vi "Create PUBREC Packet.vi"(5 "PUBREC in":refnum<class "PUBREC.lvclass">, 8 "error in (no error)":errorcluster, 9 "Packet ID":u16 format="%04x") -> (0 "error out":errorcluster, 2 "Bytes Stream":u8[](array[numeric]) format="%08b", 3 "PUBREC out":refnum<class "PUBREC.lvclass">)   [LabVIEW 2013, in "MQTT_Control_Packets.lvlib" / "PUBREC.lvclass"]
uses:
  PUBREC.lvclass
  ControlPacket/ControlPacket.lvclass/ControlPacket.ctl
  ControlPacket/ControlPacket.lvclass
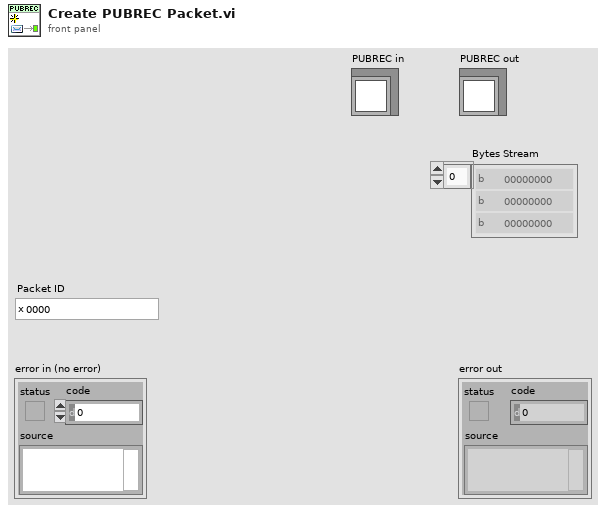
[diagram p1: front panel]
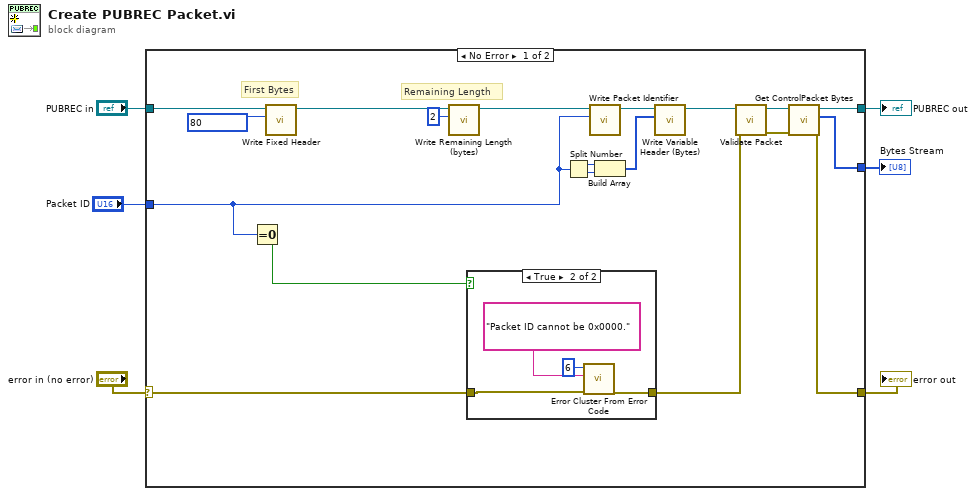
[diagram p0: block diagram]
diagram:
  n1 = case shown="No Error" "error in (no error)" {
    selector: "error in (no error)" -> [w13 w32]
    tunnel: [w9 w32] -> w3
    tunnel: [w7 w31] -> w4
    tunnel: "PUBREC in" -> [w25 w31]
    tunnel: "Packet ID" -> [w15 _]
    tunnel: [w11 _] -> w1
    frame No Error {
      # "Remaining Length"
      # "First Bytes"
      n2 = Equal To 0?(x=w15) -> (x = 0?=w14:bool)
      n3 = call "Write Fixed Header.vi"("Fixed Header"=u8 80, "ControlPacket in"=w25) -> ("ControlPacket out"=w24:refnum<class "PUBREC.lvclass">)  [unwired: 9 in]
      n4 = call "Write Remaining Length (bytes).vi"("Remaining Length (bytes)"=u32 2, "ControlPacket in"=w24) -> ("ControlPacket out"=w20:refnum<class "PUBREC.lvclass">)  [unwired: 9 in]
      n5 = case shown="True" w14 {
        tunnel: w13 -> [w26 w29]
        tunnel: [w26 w30] -> w12
        frame False {
        }
        frame True {
          n6 = call <vilib>:"Error Cluster From Error Code.vi"("error in (no error)"=w29, "error message (\"\")"="Packet ID cannot be 0x0000.", "error code (0)"=6) -> ("error out"=w30:errorcluster)  [unwired: 6 in]
        }
      }
      n7 = Split Number(x=w15) -> (hi(x)=w23:u8, lo(x)=w22:u8)
      n8 = call "Write Packet Identifier.vi"("Packet Identifier"=w15, "ControlPacket in"=w20) -> ("ControlPacket out"=w19:refnum<class "PUBREC.lvclass">)  [unwired: 9 in]
      n9 = Build Array(w23, w22) -> (w21:u8[])
      n10 = call "Write Variable Header (Bytes).vi"("Variable Header (Bytes)"=w21, "ControlPacket in"=w19) -> ("ControlPacket out"=w18:refnum<class "PUBREC.lvclass">)  [unwired: 9 in]
      n11 = call "Validate Packet.vi"("error in (no error)"=w12, "ControlPacket in"=w18) -> ("error out"=w10:errorcluster, "ControlPacket out"=w8:refnum<class "PUBREC.lvclass">)  [unwired: 8 in]
      n12 = call "Get ControlPacket Bytes.vi"("error in (no error)"=w10, "ControlPacket"=w8) -> ("error out"=w9:errorcluster, "Bytes Stream"=w11:u8[], "ControlPacket dup"=w7:refnum<class "PUBREC.lvclass">)  [unwired: 6 in, 1 out]
    }
    frame Error {
    }
  }
  "error out" <- w3
  "PUBREC out" <- w4
  "Bytes Stream" <- w1
